vi "LHF.DB.Mongo.Util.ListCollection.vi"(6 "$match":string, 8 "error in (no error)":errorcluster, 9 "fields":string[](array[string]), 10 "Collection":string, 11 "LHF.DB.Mongo in":refnum<class "LHF.DB.Mongo.lvclass">) -> (0 "error out":errorcluster, 2 "Documents":string[](array[string]), 3 "LHF.DB.Mongo out":refnum<class "LHF.DB.Mongo.lvclass">, 5 "ObjectIDs":string[](array[string]))   [LabVIEW 2013, in "LHF.DB.Mongo.lvclass"]
uses:
  LHF.DB.Mongo.lvclass
  C:/Users/schim/Desktop/Projetos/LabVIEW-MongoDB/src/Driver/MongoDB.Driver.dll
  Driver/MongoDB.Driver.dll
  C:/Users/schim/Desktop/Projetos/LabVIEW-MongoDB/src/Driver/MongoDB.Bson.dll
  Driver/MongoDB.Bson.dll
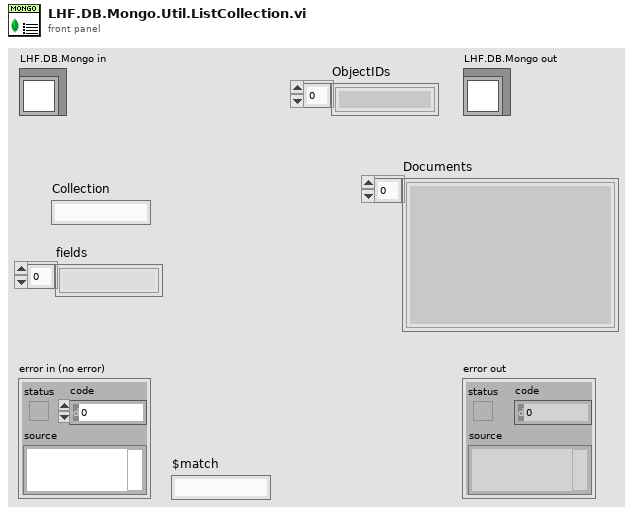
[diagram p1: front panel]
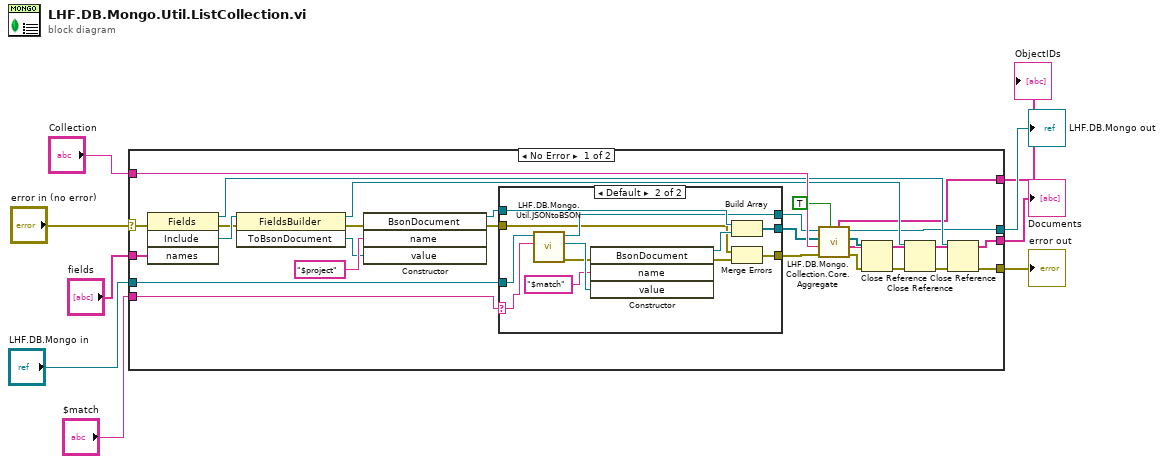
[diagram p0: block diagram]
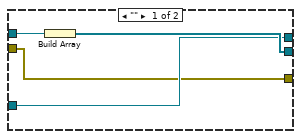
[diagram p2: hidden frame]
diagram:
  n1 = case shown="No Error" "error in (no error)" {
    selector: "error in (no error)" -> [w18 w53]
    tunnel: [w15 w53] -> w8
    tunnel: [w14 w52] -> w6
    tunnel: "LHF.DB.Mongo in" -> [w29 w52]
    tunnel: "Collection" -> [w35 _]
    tunnel: "fields" -> [w31 _]
    tunnel: "$match" -> [w12 _]
    tunnel: [w13 _] -> w2
    tunnel: [w10 _] -> w1
    frame No Error {
      n2 = invoke class="Fields" method="Include"(error in=w18, "names"=w31) -> (reference out=w28:refnum<k24>, error out=w20:errorcluster, "Include"=w33:refnum<k24>)  [unwired: 2 in, 1 out]
      n3 = invoke class="FieldsBuilder" method="ToBsonDocument"(reference=w33, error in=w20) -> (reference out=w27:refnum<k24>, error out=w19:errorcluster, "ToBsonDocument"=w32:refnum<k24>)  [unwired: 1 in]
      n4 = constructor class="BsonDocument"(error in=w19, "name"="$project", "value"=w32) -> (reference out=w30:refnum<k24>, error out=w16:errorcluster)  [unwired: 2 in, 3 out]
      n5 = case shown="Default" w12 {
        selector: w12 -> [_ w40]
        tunnel: w30 -> [w39 w49]
        tunnel: w29 -> [w37 w47]
        tunnel: [w38 w46] -> w26
        tunnel: [w37 w45] -> w25
        tunnel: [w36 w43] -> w17
        tunnel: w16 -> [w36 w41]
        frame "" {
          n6 = Build Array(w39) -> (w38:refnum<k24>[])
        }
        frame Default {
          n7 = call "LHF.DB.Mongo.Util.JSONtoBSON.vi"("JSON data"=w40, "LHF.DB.Mongo in"=w47) -> ("error out"=w44:errorcluster, "BsonDocument"=w51:refnum<k24>, "LHF.DB.Mongo out"=w45:refnum<class "LHF.DB.Mongo.lvclass">)  [unwired: 7 in]
          n8 = constructor class="BsonDocument"(error in=w44, "name"="$match", "value"=w51) -> (reference out=w48:refnum<k24>, error out=w42:errorcluster)  [unwired: 2 in, 3 out]
          n9 = Build Array(w49, w48) -> (w46:refnum<k24>[])
          n10 = Merge Errors(w41, w42) -> (w43:errorcluster)
        }
      }
      n11 = call "LHF.DB.Mongo.Collection.Core.Aggregate.vi"("Extract ObjectID"=TRUE ("Extract _id"), "error in (no error)"=w17, "Collection"=w35, "operations"=w26, "LHF.DB.Mongo in"=w25) -> ("error out"=w23:errorcluster, "Documents"=w13:string[], "operations out"=w24:refnum<k24>[], "LHF.DB.Mongo out"=w14:refnum<class "LHF.DB.Mongo.lvclass">, "ObjectID"=w10:string[])  [unwired: 2 in]
      n12 = Close Reference(reference=w24, error in (no error)=w23) -> (error out=w22:errorcluster)
      n13 = Close Reference(reference=w27, error in (no error)=w22) -> (error out=w21:errorcluster)
      n14 = Close Reference(reference=w28, error in (no error)=w21) -> (error out=w15:errorcluster)
    }
    frame Error {
    }
  }
  "error out" <- w8
  "LHF.DB.Mongo out" <- w6
  "Documents" <- w2
  "ObjectIDs" <- w1
